vi "Keithley 6487 Voltage Source.vi"(2 "error in (no error)":errorcluster, 3 "Voltage":dbl, 4 "VISA resource name":refnum<visa-resource-name>) -> (0 "error out":errorcluster, 1 "VISA resource name out":refnum<visa-resource-name>)   [LabVIEW 2020]
panel:
  in  "Source Initial Conditions":string=":SOUR:VOLT:RANG 50;:SOUR:VOLT:ILIM 2.5E-3;:SOUR:VOLT:STAT 1;"
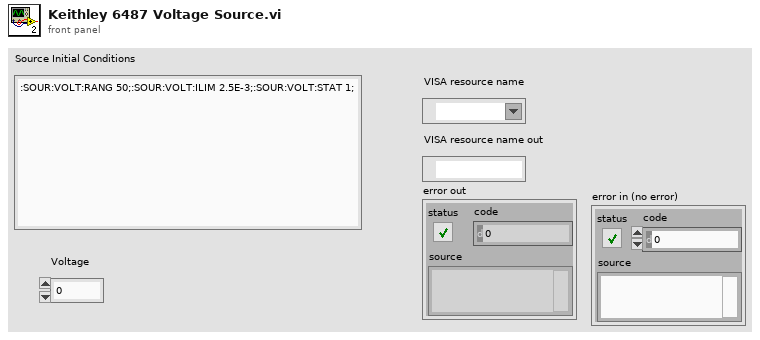
[diagram p1: front panel]
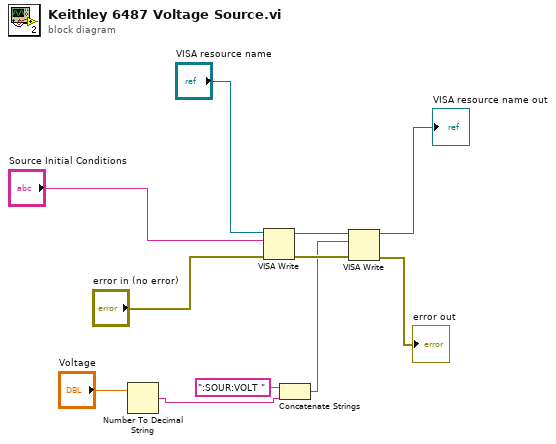
[diagram p0: block diagram]
diagram:
  n1 = Number To Decimal String(number="Voltage") -> (decimal integer string=w6:string)  [unwired: 1 in]
  n2 = VISA Write(VISA resource name="VISA resource name", write buffer="Source Initial Conditions", error in (no error)="error in (no error)") -> (VISA resource name out=w9:refnum<visa-resource-name>, error out=w10:errorcluster)  [unwired: 1 out]
  n3 = Concatenate Strings(":SOUR:VOLT " ("string"), w6) -> (w5:string)
  n4 = VISA Write(VISA resource name=w9, write buffer=w5, error in (no error)=w10) -> (VISA resource name out=→"VISA resource name out":refnum<visa-resource-name>, error out=→"error out":errorcluster)  [unwired: 1 out]
